vi "Safety systems data.vi"(7 "Arm System Status":bool, 8 "safety system raw data":string) -> (0 "Laser 2":bool, 1 "Safety System 2":bool[](array[boolean]), 2 "Laser 1":bool, 3 "Safety System 1":bool[](array[boolean]))   [LabVIEW 2020]
panel:
  out "number":u32
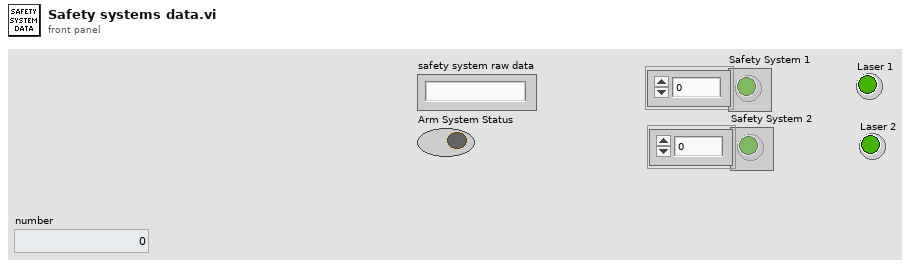
[diagram p1: front panel]
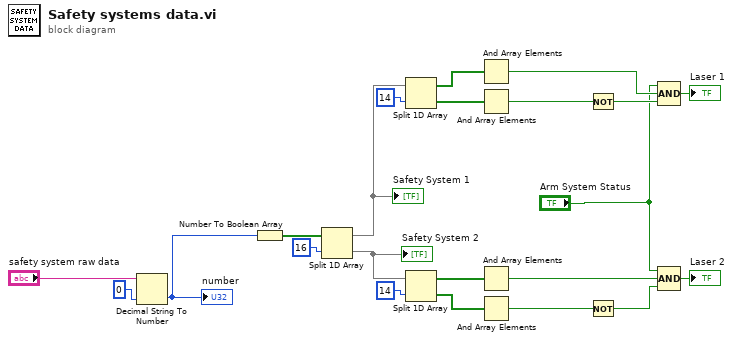
[diagram p0: block diagram]
diagram:
  n1 = Decimal String To Number(string="safety system raw data", default (0L)=u32 0) -> (number=w22:u32)  [unwired: 1 in, 1 out]
  "number" <- w22
  n2 = Number To Boolean Array(number=w22) -> (Boolean array=w20:bool[])
  n3 = Split 1D Array(array=w20, index=16) -> (first subarray=w15:bool[], second subarray=w16:bool[])
  "Safety System 1" <- w15
  "Safety System 2" <- w16
  n4 = Split 1D Array(array=w15, index=14 ("length")) -> (first subarray=w14:bool[], second subarray=w9:bool[])
  n5 = Split 1D Array(array=w16, index=14 ("length")) -> (first subarray=w13:bool[], second subarray=w12:bool[])
  n6 = And Array Elements(Boolean array=w14) -> (logical AND=w7:bool)
  n7 = And Array Elements(Boolean array=w9) -> (logical AND=w10:bool)
  n8 = And Array Elements(Boolean array=w13) -> (logical AND=w5:bool)
  n9 = And Array Elements(Boolean array=w12) -> (logical AND=w11:bool)
  n10 = Not(x=w10) -> (.not. x?=w8:bool)
  n11 = Not(x=w11) -> (.not. x?=w6:bool)
  n12 = Compound Arithmetic op=AND("Arm System Status", w7, w8) -> (→"Laser 1":bool)
  n13 = Compound Arithmetic op=AND("Arm System Status", w5, w6) -> (→"Laser 2":bool)
